vi "Close Device Driver.vi"(8 "error in (no error)":errorcluster, 11 "IVI_Counter in":refnum<class "IVI_Counter.lvclass">) -> (0 "error out":errorcluster, 3 "IVI_Counter out":refnum<class "IVI_Counter.lvclass">)   [LabVIEW 2013, in "IVI_Counter.lvlib" / "IVI_Counter.lvclass"]
doc: "Close device driver connection."
uses:
  IVI_Counter.lvclass
  Core/Actors/CS++DeviceActor/CS++DeviceActor.lvclass
  IVI_Counter.lvclass/IVI_Counter.ctl
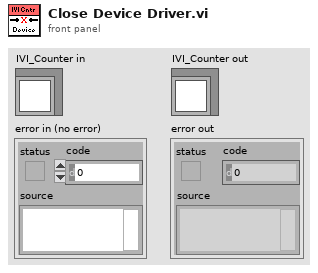
[diagram p1: front panel]
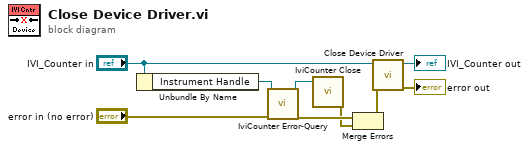
[diagram p0: block diagram]
diagram:
  n1 = Unbundle By Name("IVI_Counter in") -> ("Instrument Handle"=w6:refnum<k15>)
  n2 = call <vilib>:"IviCounter Error-Query.vi"("error in (no error)"="error in (no error)", "instrument handle"=w6) -> ("error out"=w3:errorcluster, "instrument handle out"=w5:refnum<k15>)  [unwired: 6 in, 2 out]
  n3 = call <vilib>:"IviCounter Close.vi"("instrument handle"=w5) -> ("error out"=w2:errorcluster)  [unwired: 10 in]
  n4 = Merge Errors(w3, w2) -> (w1:errorcluster)
  n5 = call-parent "Close Device Driver.vi"("error in (no error)"=w1, "CS++DeviceActor in"="IVI_Counter in") -> ("error out"=→"error out":errorcluster, "CS++DeviceActor out"=→"IVI_Counter out":refnum<class "IVI_Counter.lvclass">)  [unwired: 8 in]
